vi "指令#号分段.vi"(11 "指令输入":string) -> (2 "有匹配？":bool, 3 "分段参数":string[](array[string]))   [LabVIEW 2013]
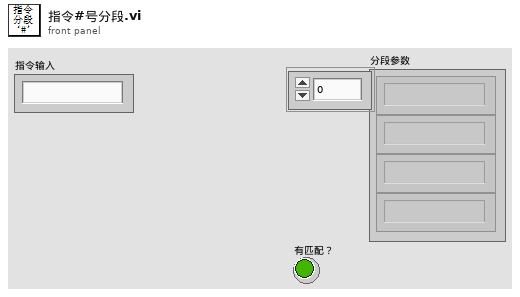
[diagram p1: front panel]
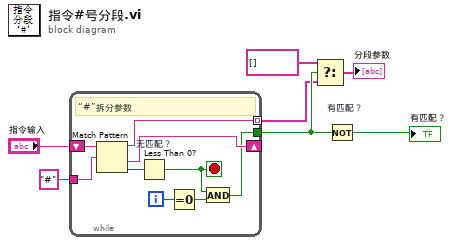
[diagram p0: block diagram]
diagram:
  n1 = while {
    tunnel: "#" ("正则表达式") -> [w15]
    shift-right: [w14] -> _
    shift-left: "指令输入" -> [w16]
    tunnel: [w13] -> w2 mode=indexing
    tunnel: [w8] -> w5
    i -> [w11]
    stop <- w10 stop-if-true
    # "“#”拆分参数"
    n2 = Match Pattern ("终端类型")(string=w16, regular expression=w15) -> (before substring=w13:string, after substring=w14:string, offset past match=w12:i32)  [unwired: 1 in, 1 out]
    n3 = Less Than 0? "无匹配？"(x=w12) -> (x < 0?=w10:bool)
    n4 = Equal To 0?(x=w11) -> (x = 0?=w9:bool)
    n5 = And(x=w10, y=w9) -> (x .and. y?=w8:bool)
  }
  n6 = Select(t=string[] [] ("分段参数"), s=w5, f=w2) -> (s? t:f=→"分段参数":string[])
  n7 = Not "有匹配？"(x=w5) -> (.not. x?=→"有匹配？":bool)
